vi "Delete product.vi"(10 "String":string, 11 "Module Number  2":dbl=1.0) -> (0 "error out":errorcluster, 2 "subarray":string[](array[string]), 3 "Sucess ?":bool)   [LabVIEW 2015, in "Copy of Untitled Library 1.lvlib"]
uses:
  Copy of Untitled Library 1.lvlib
  Controls/Caller Queue Control .ctl
  Controls/Control 1.ctl
  Controls/Enum Constant.ctl
  <userlib>/origin_lib_main/db_interface/DB Operations Enum.ctl
  <userlib>/origin_lib_main/ui_msg_lib/CTRL/Display MSG Types.ctl
  <userlib>/origin_lib_main/db_interface/DB Interface.lvlib
  <userlib>/origin_lib_main/ui_msg_lib/MSG Library.lvlib
panel:
  in  "Cluster":T1
  in  "error in (no error) 5":errorcluster
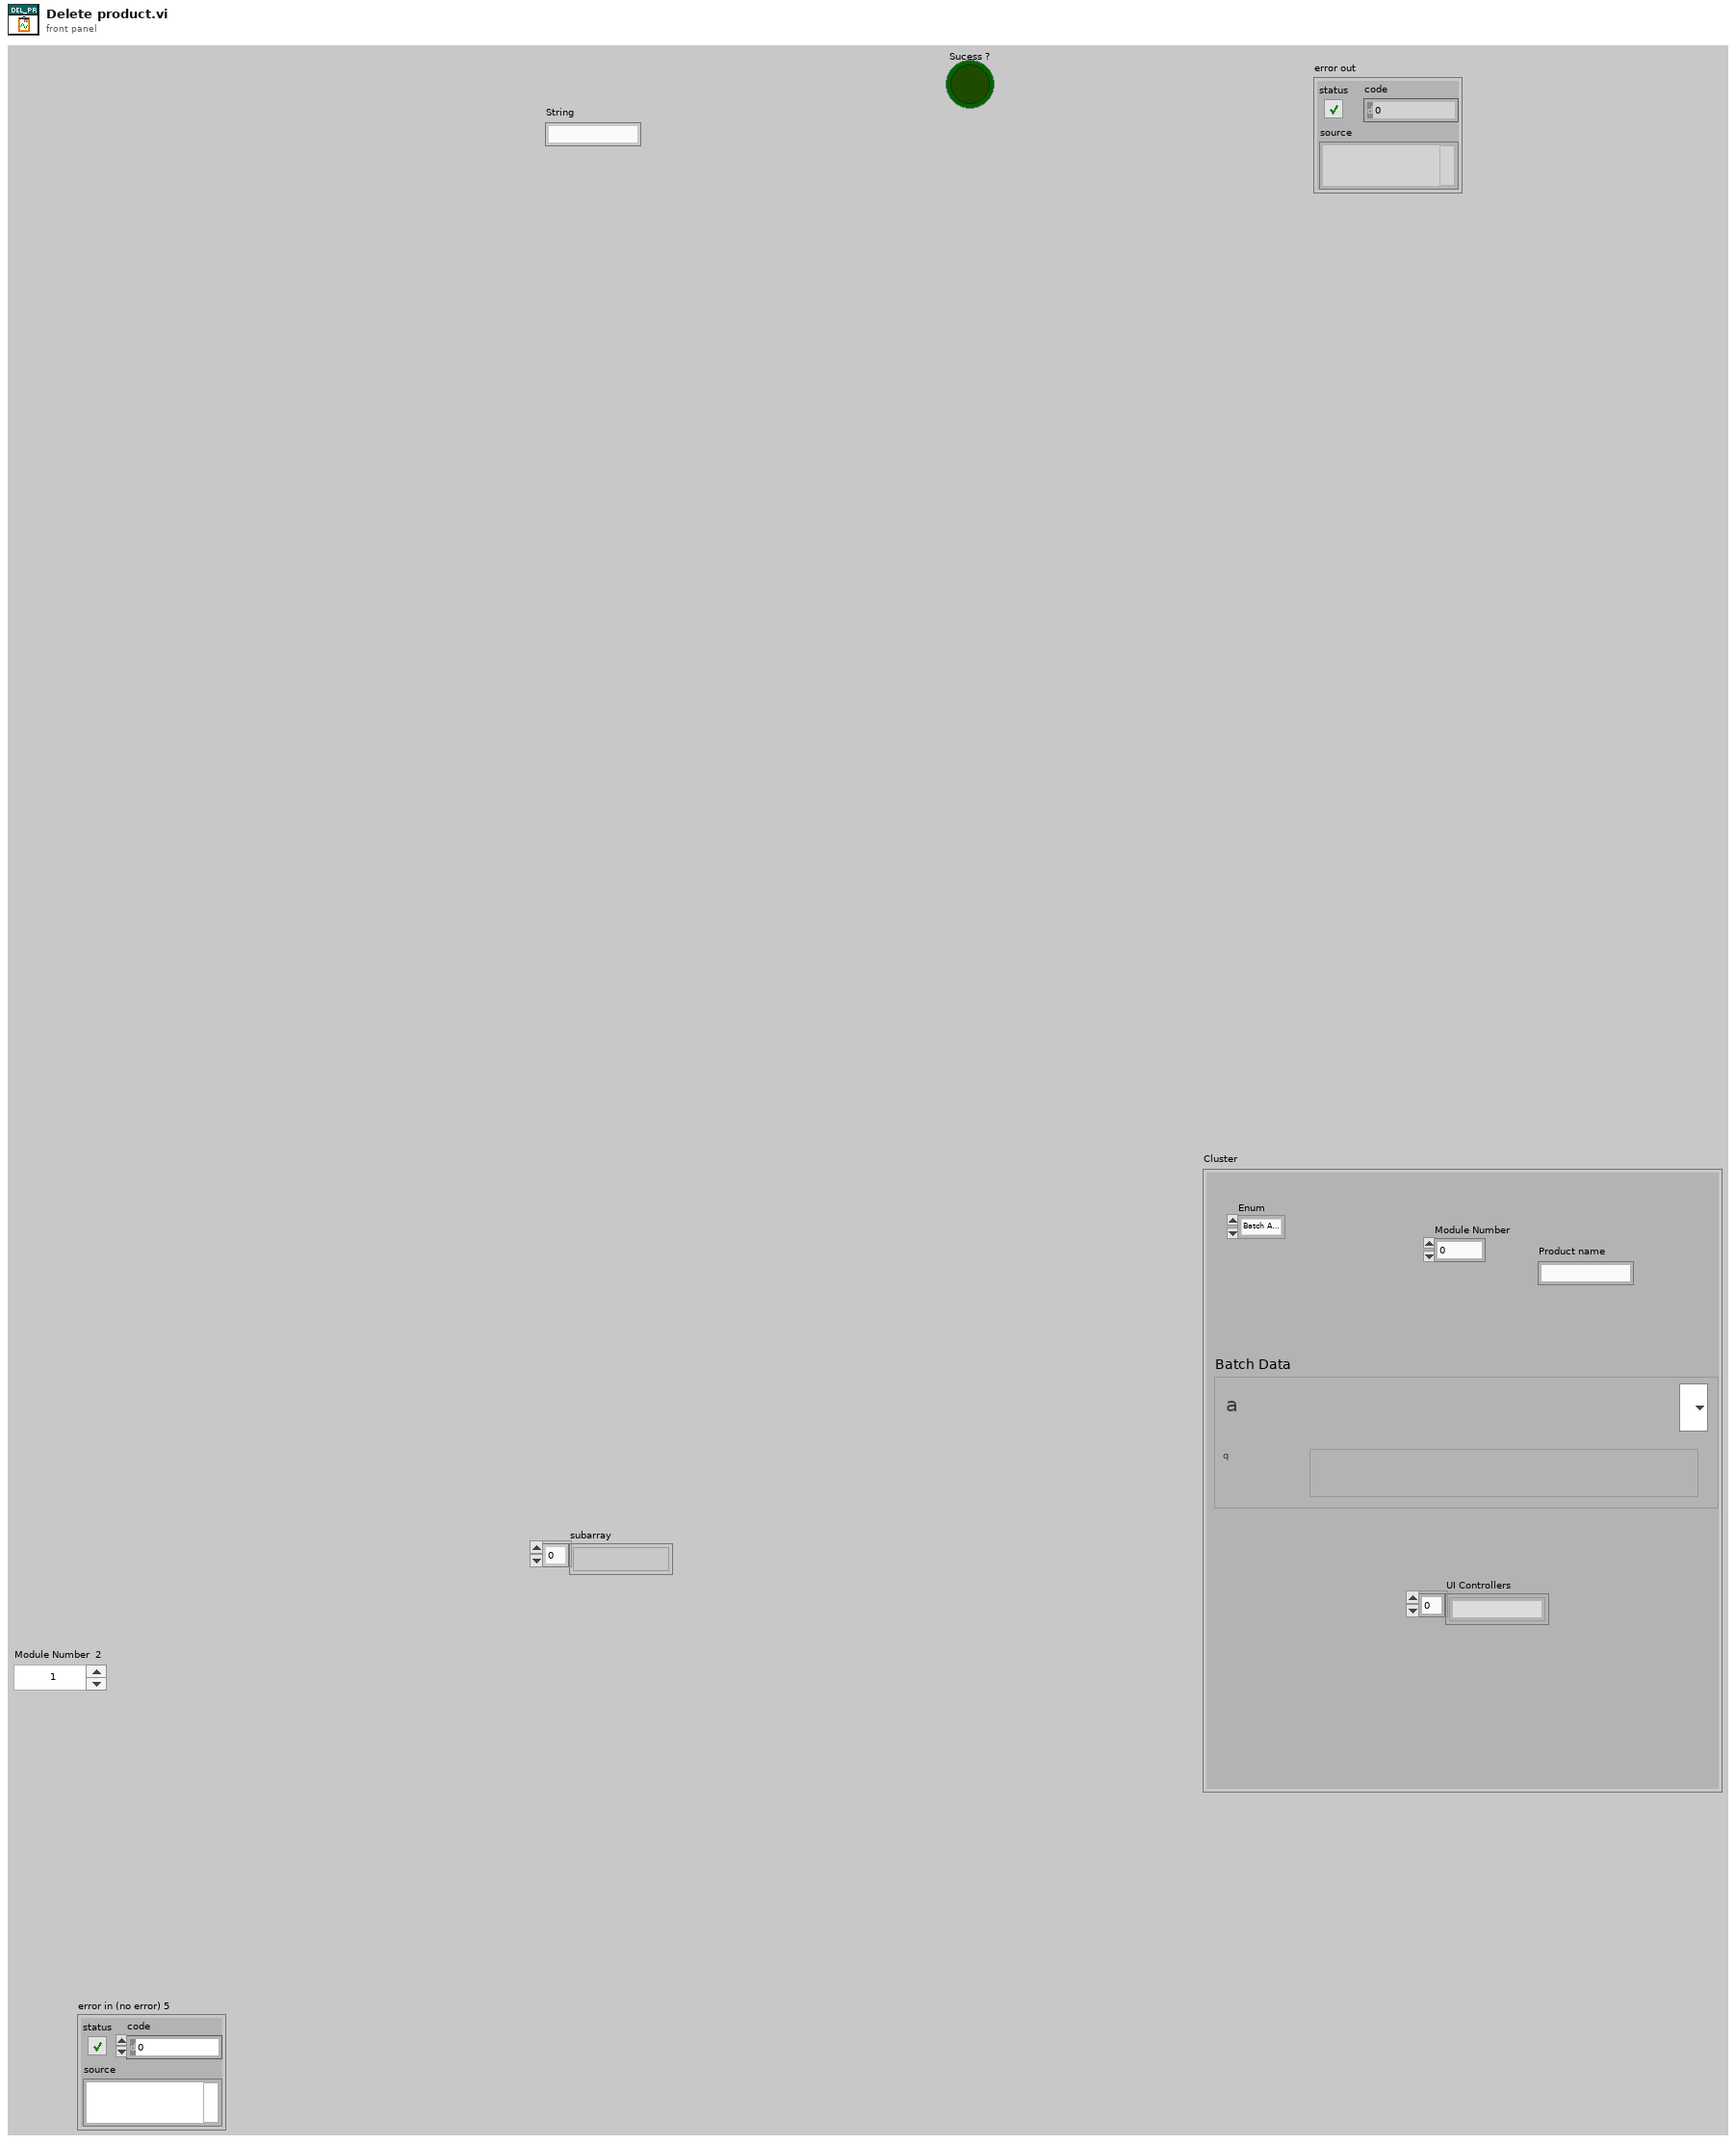
[diagram p1: front panel]
types:
  T1 = typedef "Caller Queue Control .ctl" = cluster{"Enum":enum16{"Batch Added", "Batch Deleted", "Batch Opened", "Batch Closed", "Batch Edited", "new Product Added", "Product deleted "}, "Batch Data 3":T2, "UI Controllers":string[], "Product name":string, "Module Number":dbl}
  T2 = typedef "Copy of Untitled Library 1.lvlib/Control 1.ctl" = cluster{"DATA":string, "DATA 2":string, "DATA 3":string, "DATA 4":string, "DATA 5":string, "DATA 6":string, "DATA 7":string, "DATA 8":string, "DATA 9":string, "DATA 10":string, "Product":string}
  T3 = typedef "DB Interface.lvlib/DB Operations Enum.ctl" = enum16{"Select", "Update", "Insert", "Delete", "Fetch SQL Query", "Execute SQL Query", "Drop Table", "List Tables"}
  T4 = typedef "Enum Constant.ctl" = enum16{"Init", "Read", "Write"}
  T5 = typedef "MSG Library.lvlib/Display MSG Types.ctl" = enum16{"Display MSG 1", "Display MSG 2", "Display MSG Load", "End MSG Load ", "Display 2 STR MSG"}
  T6 = typedef "FGV Data.ctl" = T7[]
  T7 = typedef "FGV Cluster Data.ctl" = cluster{"Manual/Automatic":bool, "UI Controllers ":string[], "UI Primery Key ":dbl[], "Caller Queue & MSG":T8, "Module ID":dbl, "DB Reference In":T9, "Products Columns":string[], "Cluster":cluster{"Delete Product":enum8{"Enabled", "Disabled", "Disabled and Grayed Out"}, "Add Product ":enum8{"Enabled", "Disabled", "Disabled and Grayed Out"}, "EDIT BATCH":enum8{"Enabled", "Disabled", "Disabled and Grayed Out"}, "Open Batch ":enum8{"Enabled", "Disabled", "Disabled and Grayed Out"}, "Close Batch":enum8{"Enabled", "Disabled", "Disabled and Grayed Out"}, "Delete Batch":enum8{"Enabled", "Disabled", "Disabled and Grayed Out"}, "Add Batch ":enum8{"Enabled", "Disabled", "Disabled and Grayed Out"}}}
  T8 = typedef "Queue and Caller MSG.ctl" = cluster{"Caller Queue":refnum<queue>, "Caller MSG":string}
  T9 = typedef "NI_Database_API.lvlib/Conn ObjectReference.ctl" = refnum<k1>
  T10 = enum16{"Batch Added", "Batch Deleted", "Batch Opened", "Batch Closed", "Batch Edited", "new Product Added", "Product deleted "}
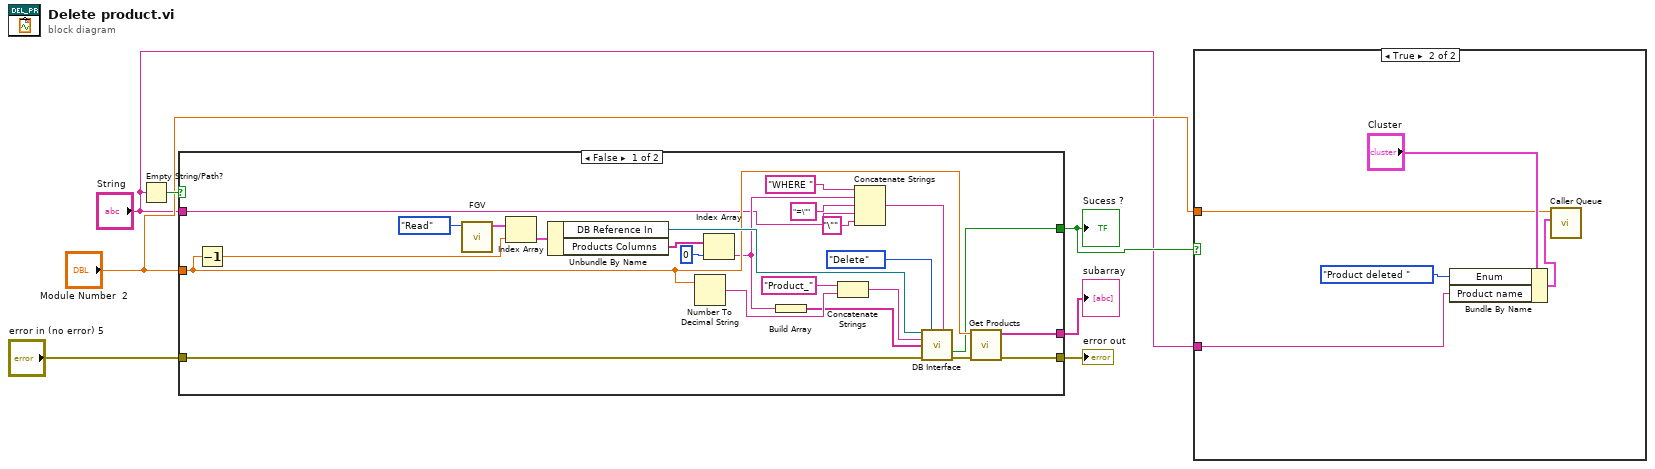
[diagram p0: block diagram]
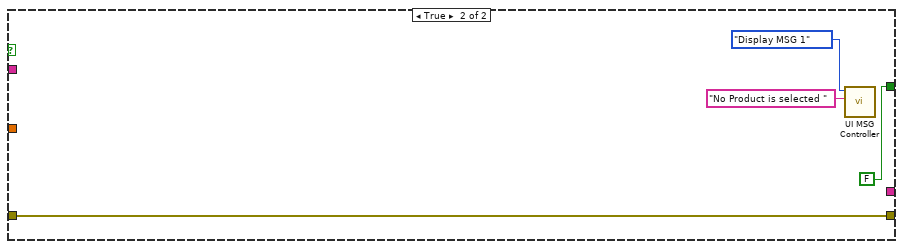
[diagram p3: hidden frame]
diagram:
  n1 = Empty String/Path?(string/path="String") -> (empty?=w5:bool)
  n2 = case shown="False" w5 {
    tunnel: [w31 w33] -> w6
    tunnel: "Module Number  2" -> [w20 _]
    tunnel: [w30 _] -> w7
    tunnel: [w15 FALSE ("Sucess ?")] -> w3
    tunnel: "String" -> [w11 _]
    tunnel: "error in (no error) 5" -> [w8 w33]
    frame False {
      n3 = Decrement(x=w20) -> (x-1=w22:dbl)
      n4 = call "FGV.vi"("Enum"=Enum_Constant."Read") -> ("Read Data"=w24:T6)  [unwired: 9 in, 1 out]
      n5 = Index Array(array=w24, index=w22) -> (element=w23:T7)
      n6 = Unbundle By Name(w23) -> ("DB Reference In"=w21:T9, "Products Columns"=w19:string[])
      n7 = Number To Decimal String(number=w20) -> (decimal integer string=w26:string)  [unwired: 1 in]
      n8 = Index Array(array=w19, index=0) -> (element=w13:string)
      n9 = Build Array(w13) -> (w17:string[])
      n10 = Concatenate Strings("Product_" ("string"), w26) -> (w25:string)
      n11 = Concatenate Strings("WHERE " ("string"), w13, "=\"" ("string"), w11, "\"" ("string")) -> (w9:string)
      n12 = call <userlib>:"DB Interface.vi"("DB Ref In"=w21, "Operation"=DB_Operations_Enum."Delete", "condition"=w9, "DB Table"=w25, "DB columns"=w17, "error in (no error)"=w8) -> ("Sucess ?"=w15:bool, "error out"=w16:errorcluster)  [unwired: 6 in, 2 out]
      n13 = call "Get Products.vi"("error in (no error) 5"=w16, "Module Number  2"=w20) -> ("error out 2"=w31:errorcluster, "subarray"=w30:string[])  [unwired: 8 in]
    }
    frame True {
      n14 = call <userlib>:"UI MSG Controller.vi"("MSG"="No Product is selected ", "Display MSG Type"=Display_MSG_Types."Display MSG 1") -> ()  [unwired: 6 in, 4 out]
    }
  }
  "error out" <- w6
  "subarray" <- w7
  "Sucess ?" <- w3
  n15 = case shown="True" w3 {
    tunnel: "Module Number  2" -> [_ w38]
    tunnel: "String" -> [_ w37]
    frame False {
    }
    frame True {
      n16 = Bundle By Name(cluster="Cluster", "Enum"=T10."Product deleted ", "Product name"=w37) -> (w36:T1)
      n17 = call "Caller Queue .vi"("Cluster"=w36, "Module Number  3"=w38) -> ()  [unwired: 9 in, 1 out]
    }
  }
